vi "Misc Timeout Counter.vi"(8 "error in (no error)":errorcluster, 10 "number of tries (3)":i32=3, 11 "counter in":i32) -> (0 "error out":errorcluster, 3 "counter out":i32)   [LabVIEW 2011, in "Misc VIs.lvlib"]
doc: "Ignores timeout error for an specified number of times (number of tries).\nAn external counter must be provided."
uses:
  Misc VIs.lvlib
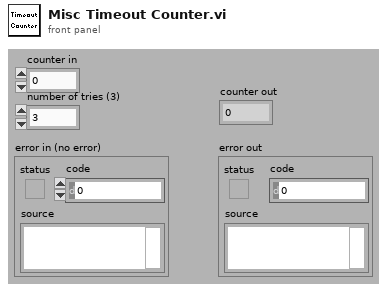
[diagram p1: front panel]
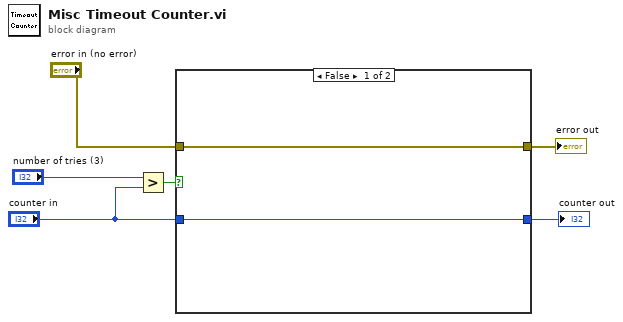
[diagram p0: block diagram]
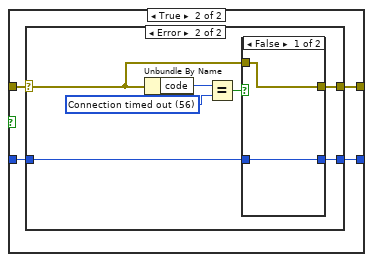
[diagram p2: hidden frame]
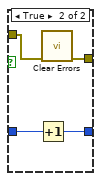
[diagram p4: hidden frame]
diagram:
  n1 = Greater?(x="number of tries (3)", y="counter in") -> (0:w5:bool)
  n2 = case shown="False" w5 {
    tunnel: "error in (no error)" -> [w8 w12]
    tunnel: [w8 w11] -> w4
    tunnel: "counter in" -> [w7 w10]
    tunnel: [w7 w9] -> w6
    frame False {
    }
    frame True {
      n3 = case shown="Error" w12 {
        selector: w12 -> [w14 w15]
        tunnel: [w14 w18] -> w11
        tunnel: w10 -> [w13 w17]
        tunnel: [w13 w16] -> w9
        frame No Error {
        }
        frame Error {
          w20 = 56 items=["No Error", "Argument Error", "Memory Full", "Out of Zone", "End of File", "File Already Open", "Generic File IO Error", "File Not Found", "File Permission Error", "Disk Full", "Duplicate Path", "Too Many Files Open", "Not Enabled", "Resource File Not Found", "Cannot Add Resource", "Resource Not Found", "Image Not Found", "Image Memory Error", "Pen Does Not Exist", "Config Bad Type", "Config Token Not Found", "Config Parse Error", "Config Memory Error", "Bad External Code Format", "Bad External Code Offset", "External Code Not Present", "Null Window", "Destroy Window Mixup", "Null Menu", "Print Aborted", "Bad Print Record", "Print Driver Error", "Windows Error During Print", "Memory Error During Print", "Print Dialog Error", "Generic Print Error", "Invalid Device Refnum", "Device Not Found", "Device Parameter Error", "Device Unit Error", "Can't Open Device", "Device Call Aborted", "Generic Error", "Cancelled By User", "Object ID Too Low", "Object ID Too High", "Object Not In Heap", "Unknown Heap", "Bad DefProc ID", "DefProc Not In Table", "Message Out Of Range", "Null Method", "Unknown Message", "Manager Call Not Supported", "Bad address", "Connection In progress", "Connection timed out", "Connection is already in progress", "Network attribute not supported", "Network error", "Address in use", "System out of memory", "Connection aborted", "Connection refused", "Connection is not connected", "Connection is already connected", "Connection closed", "Initialize error (interapplication manager)", "Bad occurrence", "Wait on unbound occurrence handler", "Occurrence queue overflow", "Bad path", "Semaphore not signaled", "Unrecognized type (interapplication manager)"] ("1st Error to Convert")
          n4 = Unbundle By Name(w15) -> ("code"=w21:i32)
          n5 = Equal?(x=w21, y=w20) -> (x = y?=w19:bool)
          n6 = case shown="False" w19 {
            tunnel: [w23 w27] -> w18
            tunnel: w17 -> [w22 w26]
            tunnel: [w22 w25] -> w16
            tunnel: w15 -> [w23 w24]
            frame False {
            }
            frame True {
              n7 = Increment(x=w26) -> (x+1=w25:i32)
              n8 = call <vilib>:"Clear Errors.vi"("error in (no error)"=w24) -> ("error out"=w27:errorcluster)  [unwired: 6 in]
            }
          }
        }
      }
    }
  }
  "counter out" <- w6
  "error out" <- w4
